vi "corerceFPGAClock.vi"(8 "error in (no error)":errorcluster, 10 "baseClock":u32 format="%.0p", 11 "requestedFrequency":dbl) -> (0 "error out":errorcluster, 2 "decimation":u16, 3 "realFrequency":dbl)   [LabVIEW 2016]
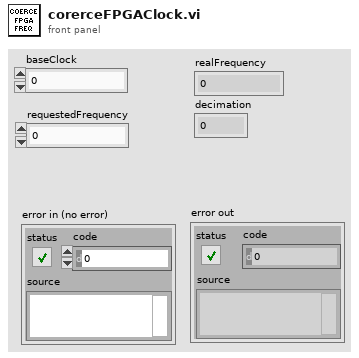
[diagram p1: front panel]
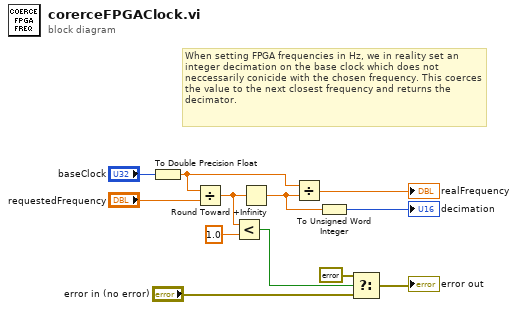
[diagram p0: block diagram]
diagram:
  # "When setting FPGA frequencies in Hz, we in reality set an integer decimation on the base clock which does not neccessarily conicide with the chosen frequency. This coerces the value to the next closest frequency and returns the decimator."
  n1 = To Double Precision Float(number="baseClock") -> (double precision float=w2:dbl)
  n2 = Divide(x=w2, y="requestedFrequency") -> (x/y=w10:dbl)
  n3 = Less?(x=w10, y=1.0) -> (x < y?=w8:bool)
  n4 = Round Toward +Infinity(x=w10) -> (ceil(x): smallest int >= x=w4:dbl)
  n5 = Divide(x=w2, y=w4) -> (x/y=→"realFrequency":dbl)
  n6 = To Unsigned Word Integer(number=w4) -> (unsigned 16bit integer=→"decimation":u16)
  n7 = Select(t=errorcluster {"status"=TRUE, "code"=0, "source"="Requested frequency smaller than base clock"}, s=w8, f="error in (no error)") -> (s? t:f=→"error out":errorcluster)
